vi "MotorWL2Pos.vi"(1 "Mono2 Center WL":dbl, 2 "HR mode":u16(ring)=3 caption="Which HR?" items=["Excitation"=1, "Detection"=2]) -> (0 "Mono2 Position":dbl)   [LabVIEW 2019]
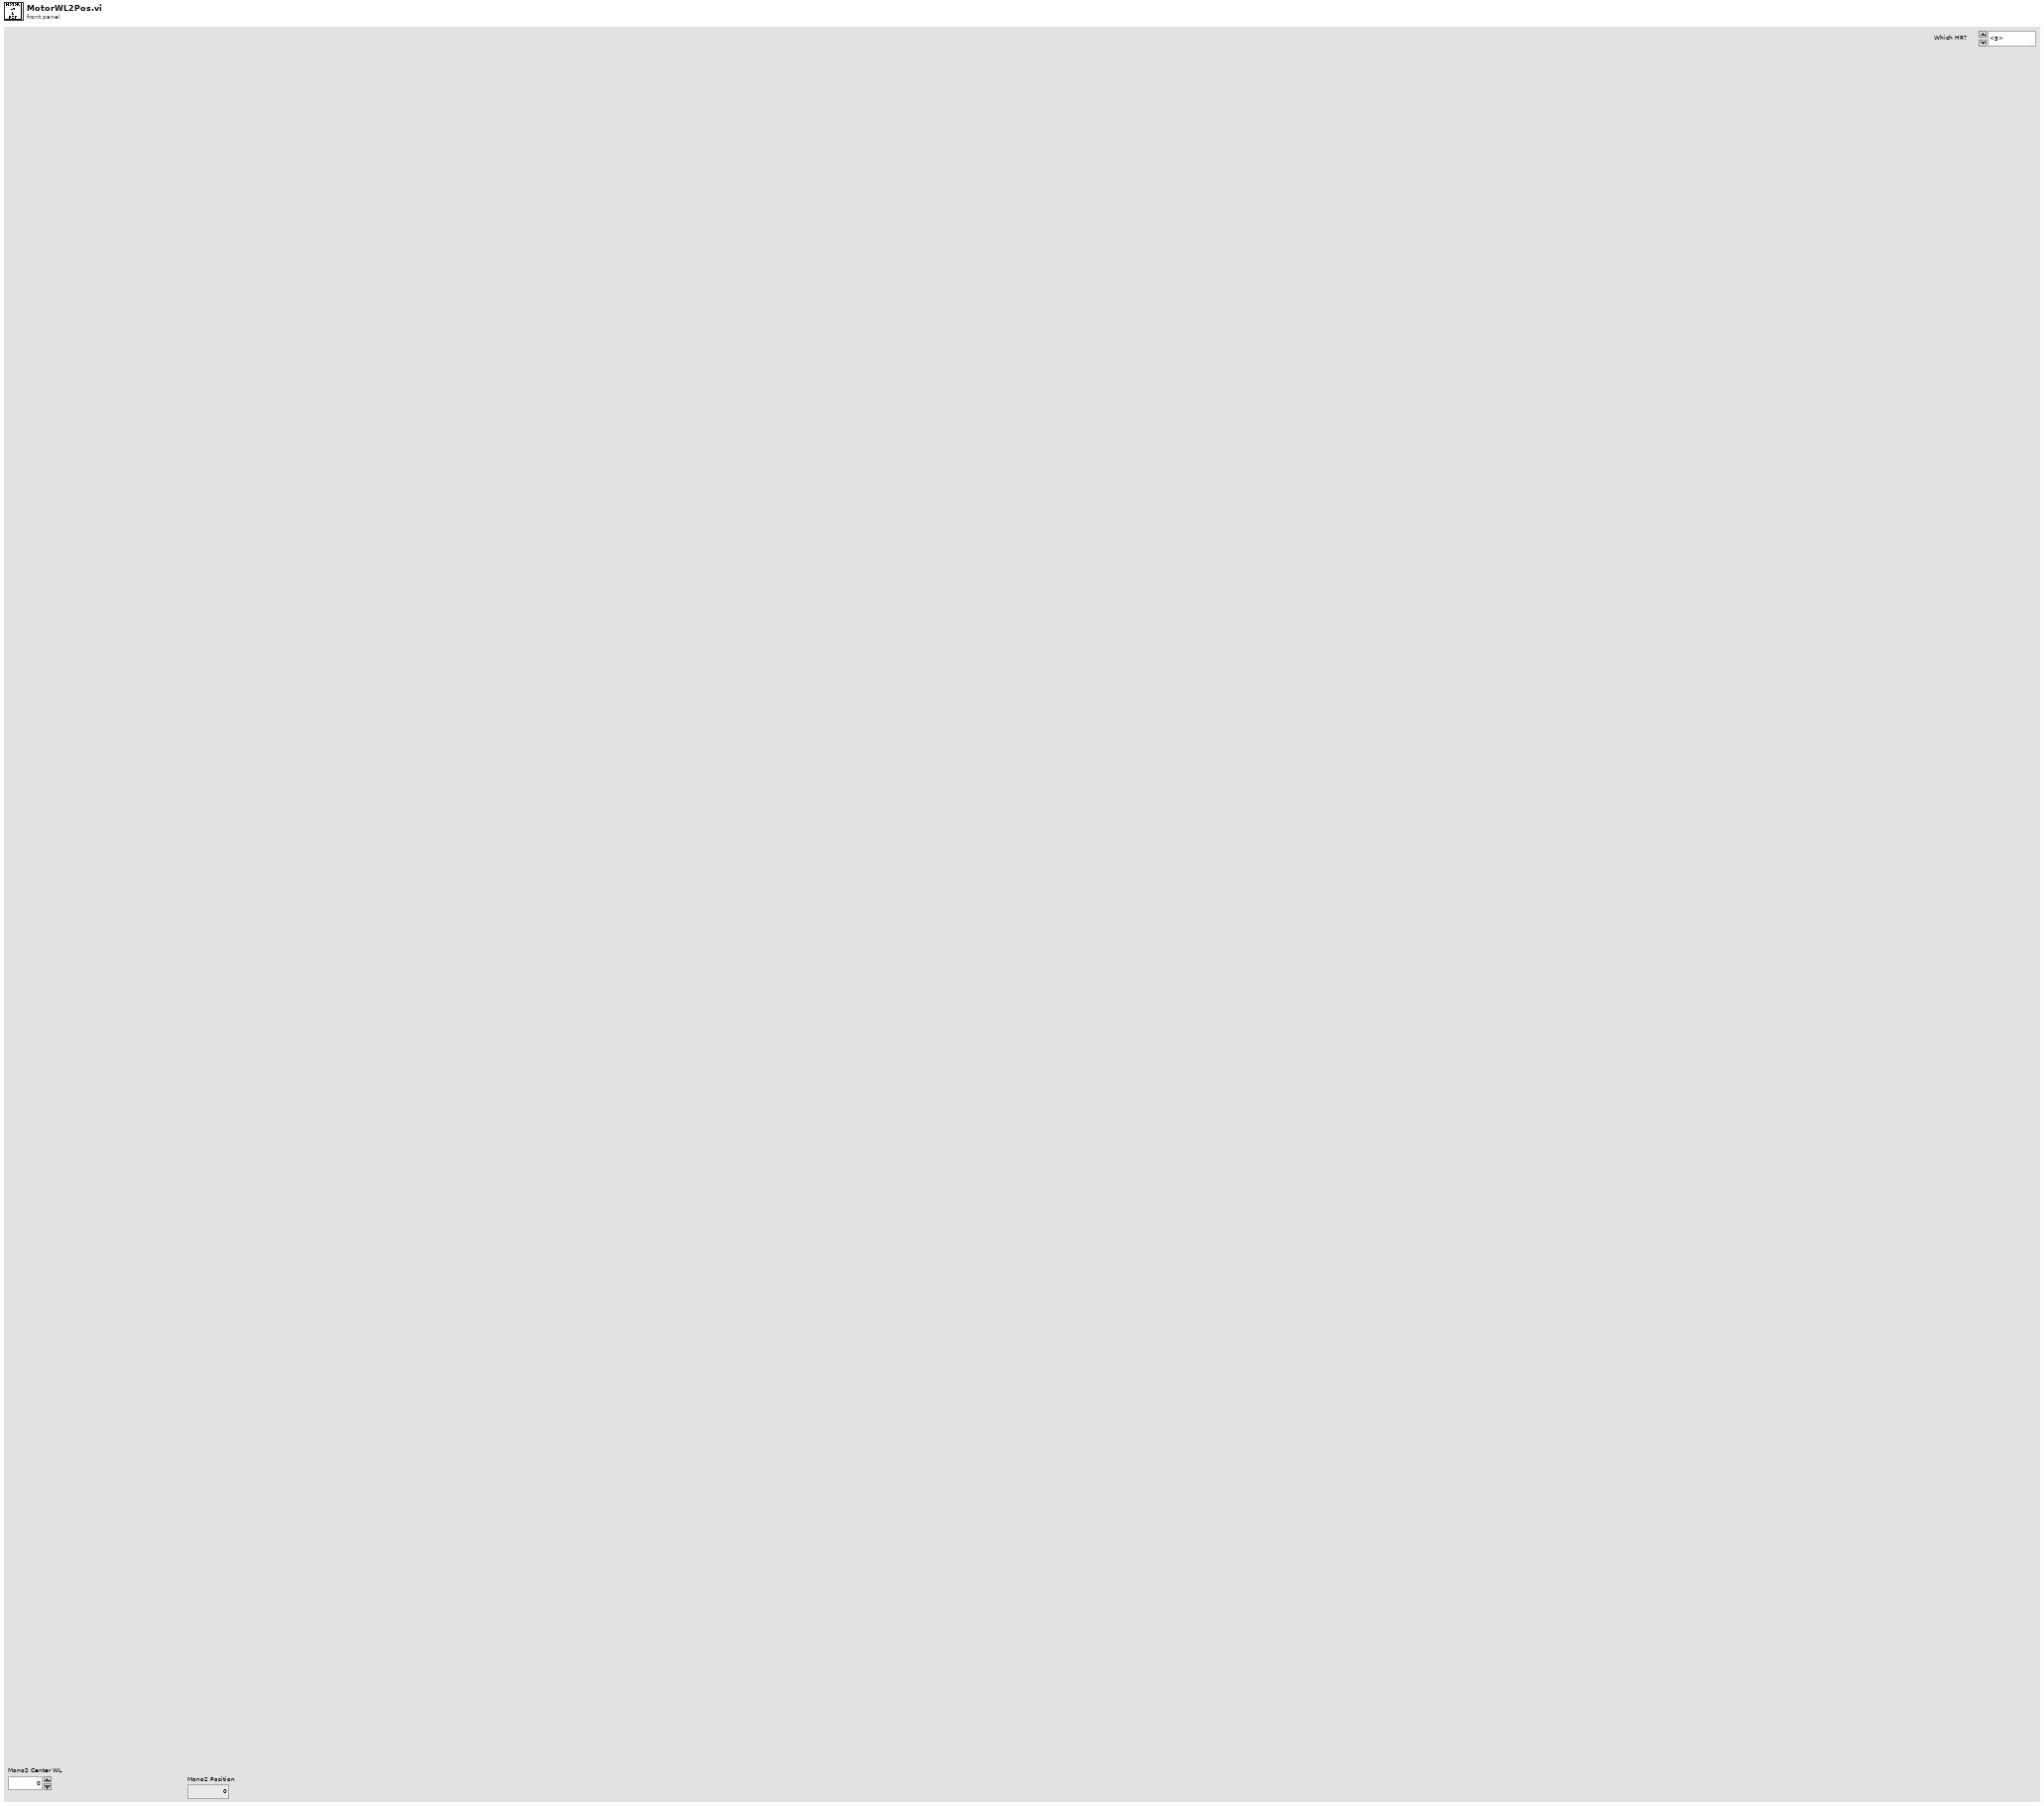
[diagram p1: front panel]
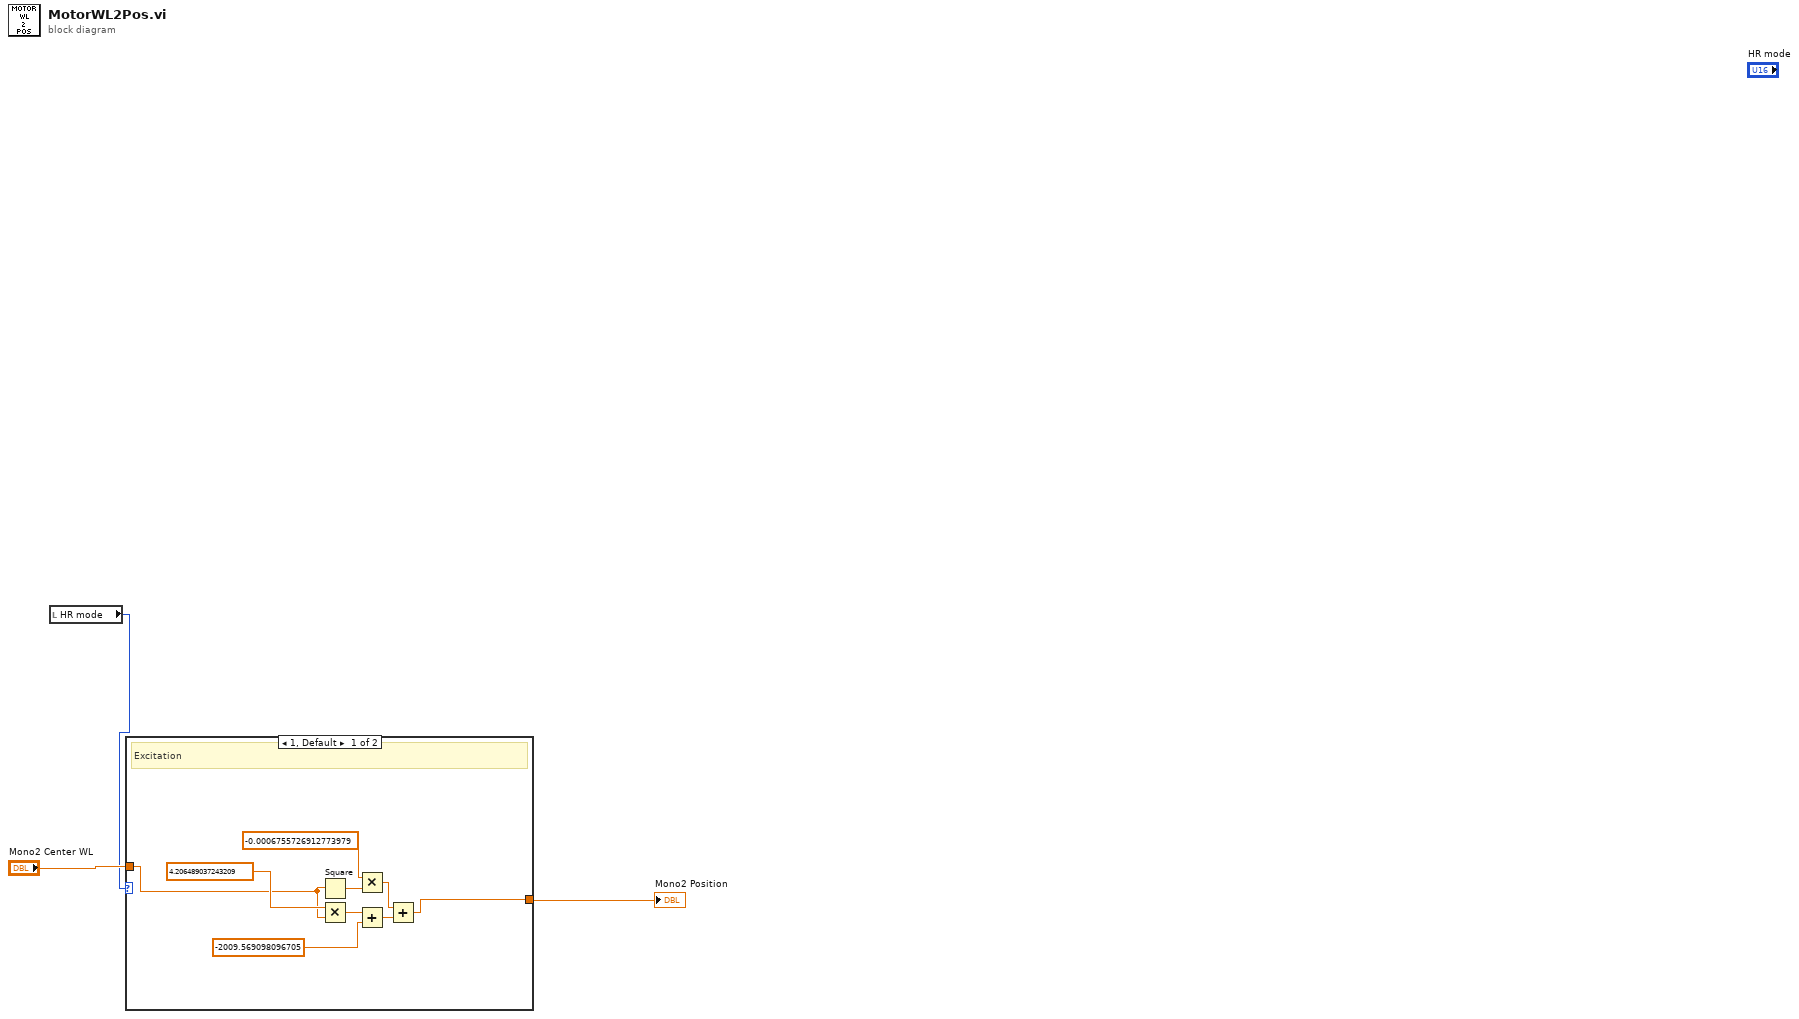
[diagram p0: block diagram]
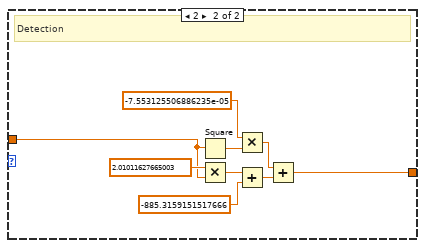
[diagram p2: hidden frame]
diagram:
  n1 = local read "HR mode"() -> (w1:u16)
  n2 = case shown="1, Default" w1 {
    tunnel: "Mono2 Center WL" -> [w4 w18]
    tunnel: [w5 w13] -> w2
    frame 1, Default {
      # "Excitation"
      n3 = Square(x=w4) -> (x^2=w11:dbl)
      n4 = Multiply(x=4.206489037243209, y=w4) -> (x*y=w12:dbl)
      n5 = Multiply(x=-0.0006755726912773979, y=w11) -> (x*y=w10:dbl)
      n6 = Add(x=w12, y=-2009.569098096705) -> (x+y=w9:dbl)
      n7 = Add(x=w10, y=w9) -> (x+y=w5:dbl)
    }
    frame 2 {
      # "Detection"
      n8 = Square(x=w18) -> (x^2=w16:dbl)
      n9 = Multiply(x=2.01011627665003, y=w18) -> (x*y=w20:dbl)
      n10 = Multiply(x=-7.553125506886235e-05, y=w16) -> (x*y=w15:dbl)
      n11 = Add(x=w20, y=-885.3159151517666) -> (x+y=w14:dbl)
      n12 = Add(x=w15, y=w14) -> (x+y=w13:dbl)
    }
  }
  "Mono2 Position" <- w2
